vi "Spurious Data Remover.vi"(9 "St Dev threshold":dbl=10.0, 11 "Cluster 1":T1={"Colour"=0, "Inst type"=enum."Pitot-static tube", "Inst name"="Manometer voltage", "Symbol"="U", "Code name"="", "Extra Info"="U", "Inst Array"=enum."PWA", "Index"=0, "Voltage Index"=0, "Extra Titles"=[], "Extra Values"=[], "Eng Values"=[], "Time (ms)"=[], "Voltage"=[], "U"=0.0, "u^2"=0.0, "u^3"=0.0, "u^4"=0.0, "Skew_u"=0.0, "Kurt_u"=0.0, "Sd Error in Mean"=0.0, "% u'/U"=0.0, "X"=0.0, "Y"=0.0, "Z"=0.0, "Spectra"={"First Name"="", "Second Name"="", "X axis name"="", "Y axis name"="", "X array"=[], "Y array"=[]}, "Autocorrelation"={"First Name"="", "Second Name"="", "X axis name"="", "Y axis name"="", "X array"=[], "Y array"=[]}, "Timescale integral to 25%"=0.0, "Sd Error in Variance"=0.0, "Calib File"=path "", "Calib Constants"=[], "Histogram"={"First Name"="", "Second Name"="", "X axis name"="", "Y axis name"="", "X array"=[], "Y array"=[]}, "Output Position"=FALSE, "Full Stats"=FALSE, "Weighting"=[]} {"Sd Error in Variance" format="%.2f"; "Skew_u" format="%.2f"; "% u'/U" format="%.2f"; "Sd Error in Mean" format="%.2f"; "Kurt_u" format="%.2f"; "u^4" format="%.2f"; "u^3" format="%.2f"; "U" format="%.2f"; "u^2" format="%.2f"}) -> (3 "Cluster 1 Spurious points removed":T1={"Colour"=0, "Inst type"=enum."Pitot-static tube", "Inst name"="Manometer voltage", "Symbol"="U", "Code name"="", "Extra Info"="U", "Inst Array"=enum."PWA", "Index"=0, "Voltage Index"=0, "Extra Titles"=[], "Extra Values"=[], "Eng Values"=[], "Time (ms)"=[], "Voltage"=[], "U"=0.0, "u^2"=0.0, "u^3"=0.0, "u^4"=0.0, "Skew_u"=0.0, "Kurt_u"=0.0, "Sd Error in Mean"=0.0, "% u'/U"=0.0, "X"=0.0, "Y"=0.0, "Z"=0.0, "Spectra"={"First Name"="", "Second Name"="", "X axis name"="", "Y axis name"="", "X array"=[], "Y array"=[]}, "Autocorrelation"={"First Name"="", "Second Name"="", "X axis name"="", "Y axis name"="", "X array"=[], "Y array"=[]}, "Timescale integral to 25%"=0.0, "Sd Error in Variance"=0.0, "Calib File"=path "", "Calib Constants"=[], "Histogram"={"First Name"="", "Second Name"="", "X axis name"="", "Y axis name"="", "X array"=[], "Y array"=[]}, "Output Position"=FALSE, "Full Stats"=FALSE, "Weighting"=[]} {"Sd Error in Variance" format="%.2f"; "Skew_u" format="%.2f"; "% u'/U" format="%.2f"; "Sd Error in Mean" format="%.2f"; "Kurt_u" format="%.2f"; "u^4" format="%.2f"; "u^3" format="%.2f"; "U" format="%.2f"; "u^2" format="%.2f"})   [LabVIEW 2011]
uses:
  Controls/Analysis_info_cluster.ctl
  Controls/Inst_type.ctl
  Controls/Instrument_Array.ctl
  Controls/XY_Plot_Cluster.ctl
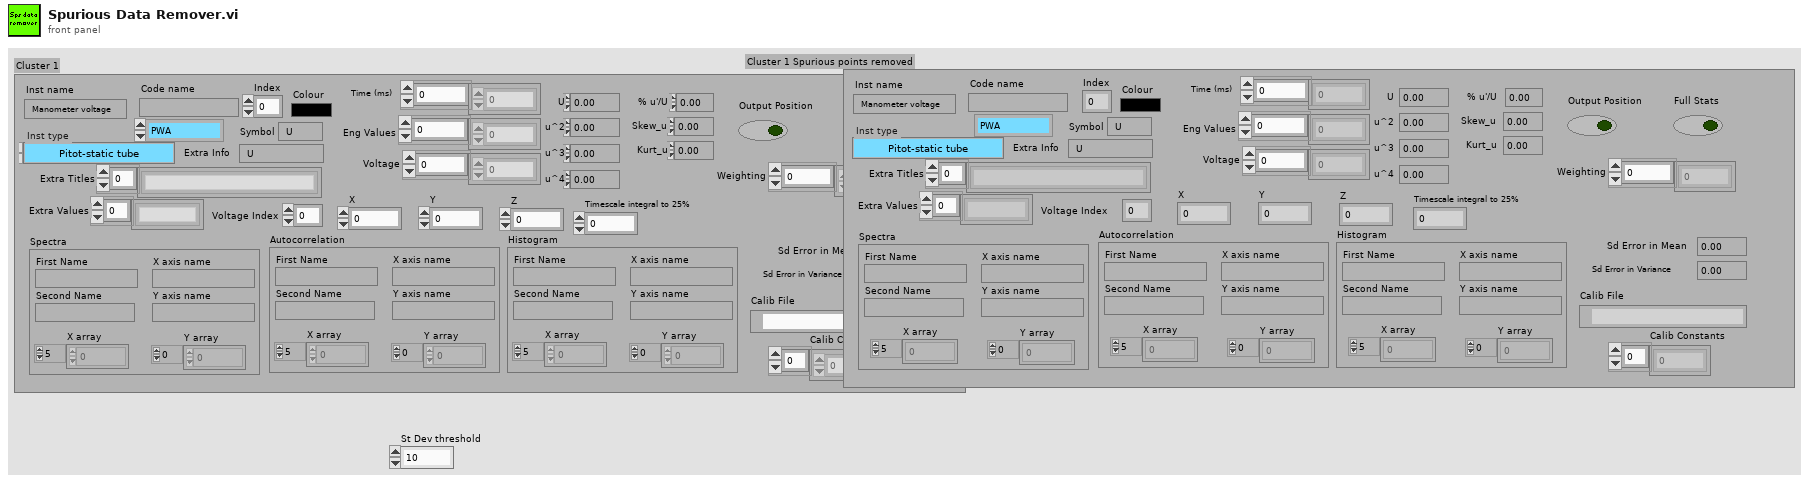
[diagram p1: front panel]
types:
  T1 = typedef "Analysis_info_cluster.ctl" = cluster{"Colour":u32, "Inst type":T2, "Inst name":string, "Symbol":string, "Code name":string, "Extra Info":string, "Inst Array":T3, "Index":i32, "Voltage Index":i32, "Extra Titles":string[], "Extra Values":string[], "Eng Values":dbl[], "Time (ms)":dbl[], "Voltage":dbl[], "U":dbl, "u^2":dbl, "u^3":dbl, "u^4":dbl, "Skew_u":dbl, "Kurt_u":dbl, "Sd Error in Mean":dbl, "% u'/U":dbl, "X":dbl, "Y":dbl, "Z":dbl, "Spectra":T4, "Autocorrelation":T4, "Timescale integral to 25%":dbl, "Sd Error in Variance":dbl, "Calib File":path, "Calib Constants":dbl[], "Histogram":T4, "Output Position":bool, "Full Stats":bool, "Weighting":dbl[]}
  T2 = typedef "Inst_type.ctl" = enum16{"Propeller anemometer", "Raw voltage", "Pressure Transducer", "Pitot-static tube", "Preston tube", "Hot wire", "Cross wire 1", "Cross wire 2", "Generic Linear", "Generic Polynomial", "Generic BackPoly", "Fast FID", "Thermocouple", "Cold wire", "Pulsed Wire", "LDA Vel", "LDA Tran time", "LDA Arr time"}
  T3 = typedef "Instrument_Array.ctl" = enum16{"PWA", "LDA", "Analogue"}
  T4 = typedef "XY_Plot_Cluster.ctl" = cluster{"First Name":string, "Second Name":string, "X axis name":string, "Y axis name":string, "X array":dbl[], "Y array":dbl[]}
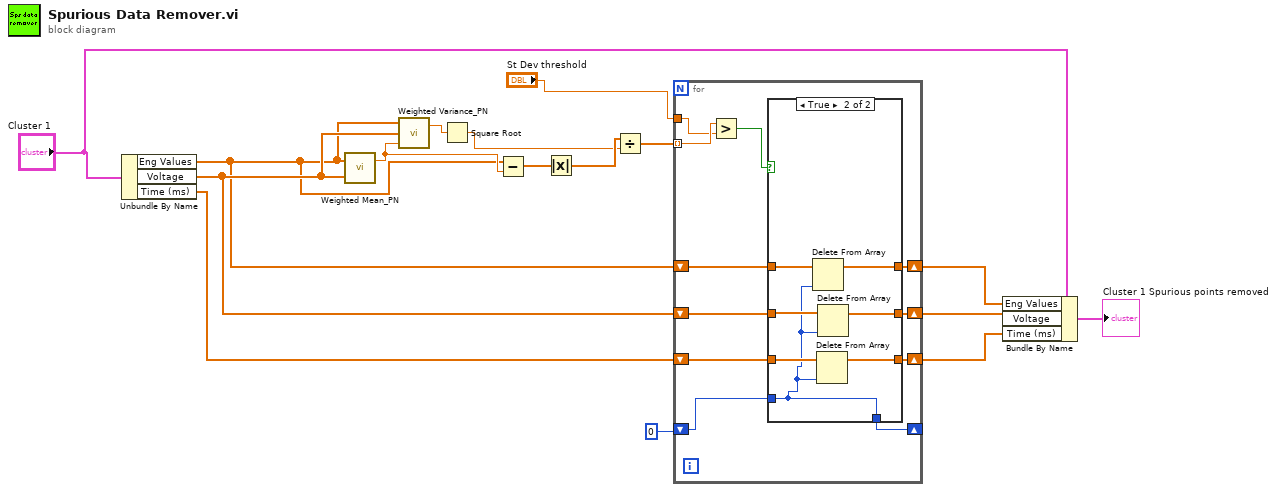
[diagram p0: block diagram]
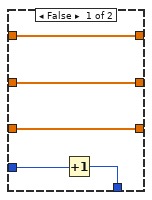
[diagram p2: hidden frame]
diagram:
  n1 = Unbundle By Name("Cluster 1") -> ("Eng Values"=w8:dbl[], "Voltage"=w9:dbl[], "Time (ms)"=w10:dbl[])
  n2 = call "Weighted Mean_PN.vi"("weights"=w9, "1D data"=w8) -> ("Weighted mean"=w15:dbl)  [unwired: 1 in]
  n3 = call "Weighted Variance_PN.vi"("Weighted mean"=w15, "weights"=w9, "1D data"=w8) -> ("Weighted variance"=w16:dbl)  [unwired: 1 in]
  n4 = Square Root(x=w16) -> (sqrt(x)=w11:dbl)
  n5 = Subtract(x=w8, y=w15) -> (x-y=w14:dbl[])
  n6 = Absolute Value(x=w14) -> (abs(x)=w13:dbl[])
  n7 = Divide(x=w13, y=w11) -> (x/y=w12:dbl[])
  n8 = for {
    tunnel: w12 -> [w27] mode=indexing
    tunnel: "St Dev threshold" -> [w26]
    shift-right: [w19] -> w5
    shift-left: w10 -> [w24]
    shift-right: [w21] -> w7
    shift-left: w8 -> [w22]
    shift-right: [w20] -> w6
    shift-left: w9 -> [w23]
    shift-right: [w17] -> _
    shift-left: 0 -> [w18]
    n9 = Greater?(x=w27, y=w26) -> (0:w25:bool)
    n10 = case shown="True" w25 {
      tunnel: w24 -> [w30 w38]
      tunnel: w23 -> [w31 w37]
      tunnel: w22 -> [w32 w39]
      tunnel: [w32 w36] -> w21
      tunnel: [w31 w35] -> w20
      tunnel: [w30 w34] -> w19
      tunnel: w18 -> [w29 w33]
      tunnel: [w28 w33] -> w17
      frame False {
        n11 = Increment(x=w29) -> (x+1=w28:i32)
      }
      frame True {
        n12 = Delete From Array(array=w39, index=w33) -> (array with subset deleted=w36:dbl[])  [unwired: 1 in, 1 out]
        n13 = Delete From Array(array=w38, index=w33) -> (array with subset deleted=w34:dbl[])  [unwired: 1 in, 1 out]
        n14 = Delete From Array(array=w37, index=w33) -> (array with subset deleted=w35:dbl[])  [unwired: 1 in, 1 out]
      }
    }
  }
  n15 = Bundle By Name(cluster="Cluster 1", "Eng Values"=w7, "Voltage"=w6, "Time (ms)"=w5) -> (→"Cluster 1 Spurious points removed":T1)
